vi "SMTP Email Convert EUC to JIS.vi"(11 "text in":string) -> (3 "text out":string)   [LabVIEW 2011, in "NewNI_SMTPEmail.lvlib"]
uses:
  NewNI_SMTPEmail.lvlib
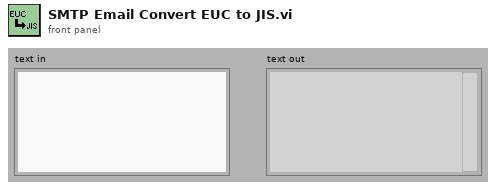
[diagram p1: front panel]
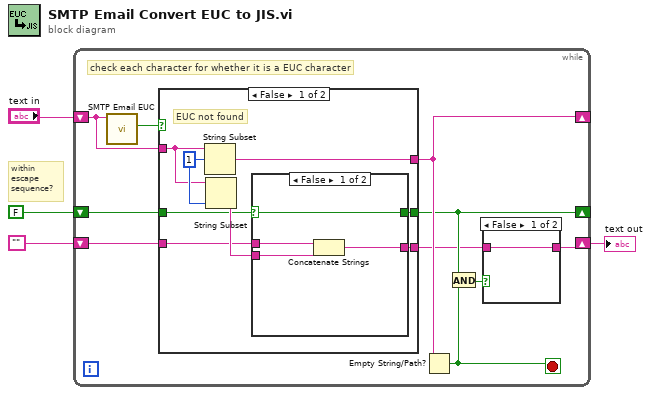
[diagram p0: block diagram]
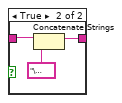
[diagram p2: hidden frame]
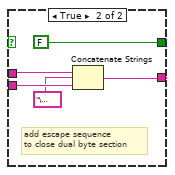
[diagram p3: hidden frame]
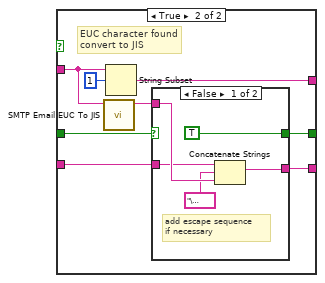
[diagram p4: hidden frame]
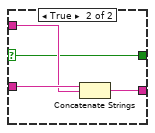
[diagram p5: hidden frame]
diagram:
  # "within\nescape\nsequence?"
  n1 = while {
    shift-right: [w12] -> _
    shift-left: "text in" -> [w6]
    shift-right: [w7] -> w1
    shift-left: "" -> [w14]
    shift-right: [w11] -> _
    shift-left: FALSE -> [w13]
    stop <- w10 stop-if-true
    # "check each character for whether it is a EUC character"
    n2 = call "SMTP Email EUC.vi"("text"=w6) -> ("isEUC?"=w5:bool)  [unwired: 10 out]
    n3 = case shown="False" w5 {
      tunnel: w6 -> [w24 w37]
      tunnel: [w23 w42] -> w12
      tunnel: w14 -> [w22 w41]
      tunnel: [w20 w40] -> w8
      tunnel: w13 -> [w21 w39]
      tunnel: [w19 w38] -> w11
      frame False {
        w26 = 1 ("offset (0)")
        # "EUC not found"
        n4 = String Subset(string=w24, offset (0)=w26) -> (substring=w23:string)  [unwired: 1 out]
        n5 = String Subset(string=w24, length (rest)=w26) -> (substring=w25:string)  [unwired: 1 out]
        n6 = case shown="False" w21 {
          selector: w21 -> [w27 _]
          tunnel: w25 -> [w30 w35]
          tunnel: w22 -> [w29 w32]
          tunnel: [w28 w34] -> w20
          tunnel: [w27 FALSE] -> w19
          frame False {
            n7 = Concatenate Strings(w29, w30) -> (w28:string)
          }
          frame True {
            # "add escape sequence\nto close dual byte section"
            n8 = Concatenate Strings(w32, "\u001b(J" ("string"), w35) -> (w34:string)
          }
        }
      }
      frame True {
        # "EUC character found\nconvert to JIS"
        n9 = call "SMTP Email EUC To JIS.vi"("text in"=w37) -> ("text out"=w36:string)  [unwired: 10 out]
        n10 = String Subset(string=w37, offset (0)=1) -> (substring=w42:string)  [unwired: 1 out]
        n11 = case shown="False" w39 {
          selector: w39 -> [_ w49]
          tunnel: w41 -> [w45 w52]
          tunnel: [w48 w51] -> w40
          tunnel: w36 -> [w47 w50]
          tunnel: [TRUE w49] -> w38
          frame False {
            # "add escape sequence\nif necessary"
            n12 = Concatenate Strings(w45, "\u001b$B" ("string"), w47) -> (w48:string)
          }
          frame True {
            n13 = Concatenate Strings(w52, w50) -> (w51:string)
          }
        }
      }
    }
    n14 = Empty String/Path?(string/path=w12) -> (empty?=w10:bool)
    n15 = And(x=w11, y=w10) -> (x .and. y?=w9:bool)
    n16 = case shown="False" w9 {
      tunnel: w8 -> [w15 w18]
      tunnel: [w15 w16] -> w7
      frame False {
      }
      frame True {
        n17 = Concatenate Strings(w18, "\u001b(J" ("string")) -> (w16:string)
      }
    }
  }
  "text out" <- w1
